vi "FTDI_MPSSE_SetChannel.vi"(8 "error in (no error)":errorcluster, 10 "config":T1={"ClockRate"=2000, "LatencyTimer"=255, "configOptions 24-31"=0, "configOptions 16-23"=0, "configOptions 8-15"=0, "configOptions 0-7"=32, "Pin"=0, "reserved"=0} {"configOptions 24-31" format="%x"; "configOptions 16-23" format="%x"; "configOptions 8-15" format="%x"; "configOptions 0-7" format="%x"}, 11 "handle":u32 format="%08x") -> (0 "error out":errorcluster, 3 "handle out":u32)   [LabVIEW 2018]
uses:
  dll/libMPSSE.dll
  libMPSSE-SPI.lvlib
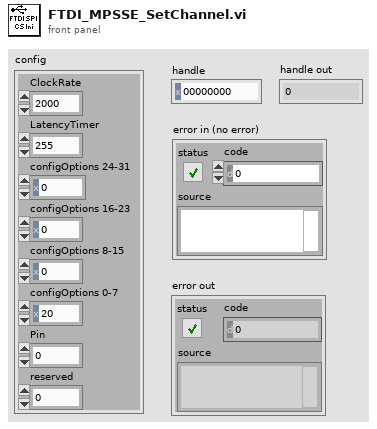
[diagram p1: front panel]
types:
  T1 = cluster{"ClockRate":u32, "LatencyTimer":u8, "configOptions 24-31":i8, "configOptions 16-23":i8, "configOptions 8-15":i8, "configOptions 0-7":u32, "Pin":u32, "reserved":u16}
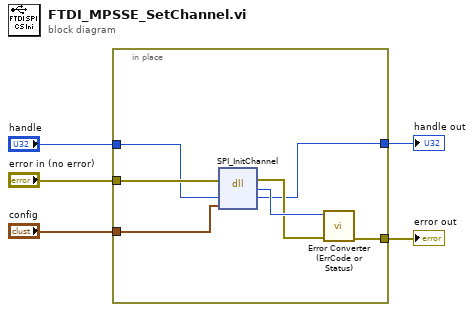
[diagram p0: block diagram]
diagram:
  n1 = in-place {
    in-place-border: "config" -> [w10]
    in-place-border: [w9] -> w4
    in-place-border: "error in (no error)" -> [w8]
    in-place-border: "handle" -> [w7]
    in-place-border: [w6] -> w1
    n2 = dll-call lib="D:/LABVIEW/SEQUENSER SNA/FTDI SPI/dll/libMPSSE.dll" fn="SPI_InitChannel"(error in=w8, "handle"=w7, "config"=w10) -> (error out=w11:errorcluster, "return type"=w12:u32, "handle"=w6:u32)  [unwired: 3 in, 1 out]
    n3 = call "Error Converter (ErrCode or Status).vi"("error in (no error)"=w11, "error code"=w12) -> ("error out"=w9:errorcluster)  [unwired: 9 in]
  }
  "error out" <- w4
  "handle out" <- w1
